vi "HexConvert.vi"(8 "E Field":string[](array[string]), 9 "Phase Field":string[](array[string]), 10 "Pockels_Galvo_Params":T1, 11 "Frequency Record":T2) -> (2 "Interrupted":bool, 3 "Hex":string)   [LabVIEW 2017]
uses:
  Controls/Frequency Record.ctl
  Controls/Pockels_Galvo_Params.ctl
  Global Variables/General Globals.vi
panel:
  out "x-y":u32
  out "Numeric":i32
  # "RE-ENTRANT"
  # "SUBROUTINE"
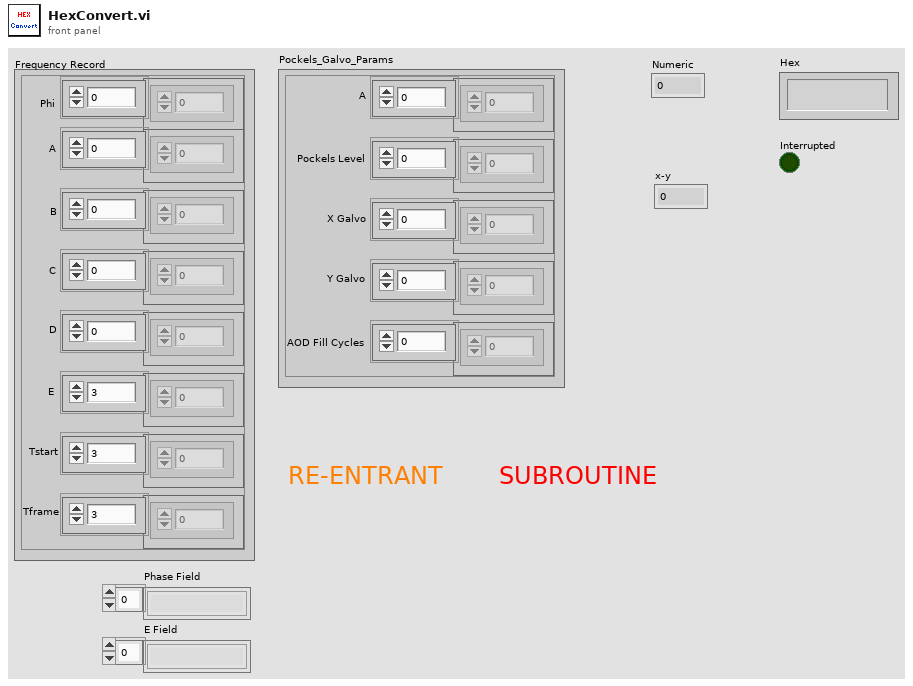
[diagram p1: front panel]
types:
  T1 = typedef "Pockels_Galvo_Params.ctl" = cluster{"A":dbl[], "Pockels Level":dbl[], "X Galvo":dbl[], "Y Galvo":dbl[], "AOD Fill Cycles":dbl[]}
  T2 = typedef "Frequency Record.ctl" = cluster{"Phi":dbl[], "A":dbl[], "B":dbl[], "C":dbl[], "D":dbl[], "E":dbl[], "Tstart":dbl[], "Tframe":dbl[]}
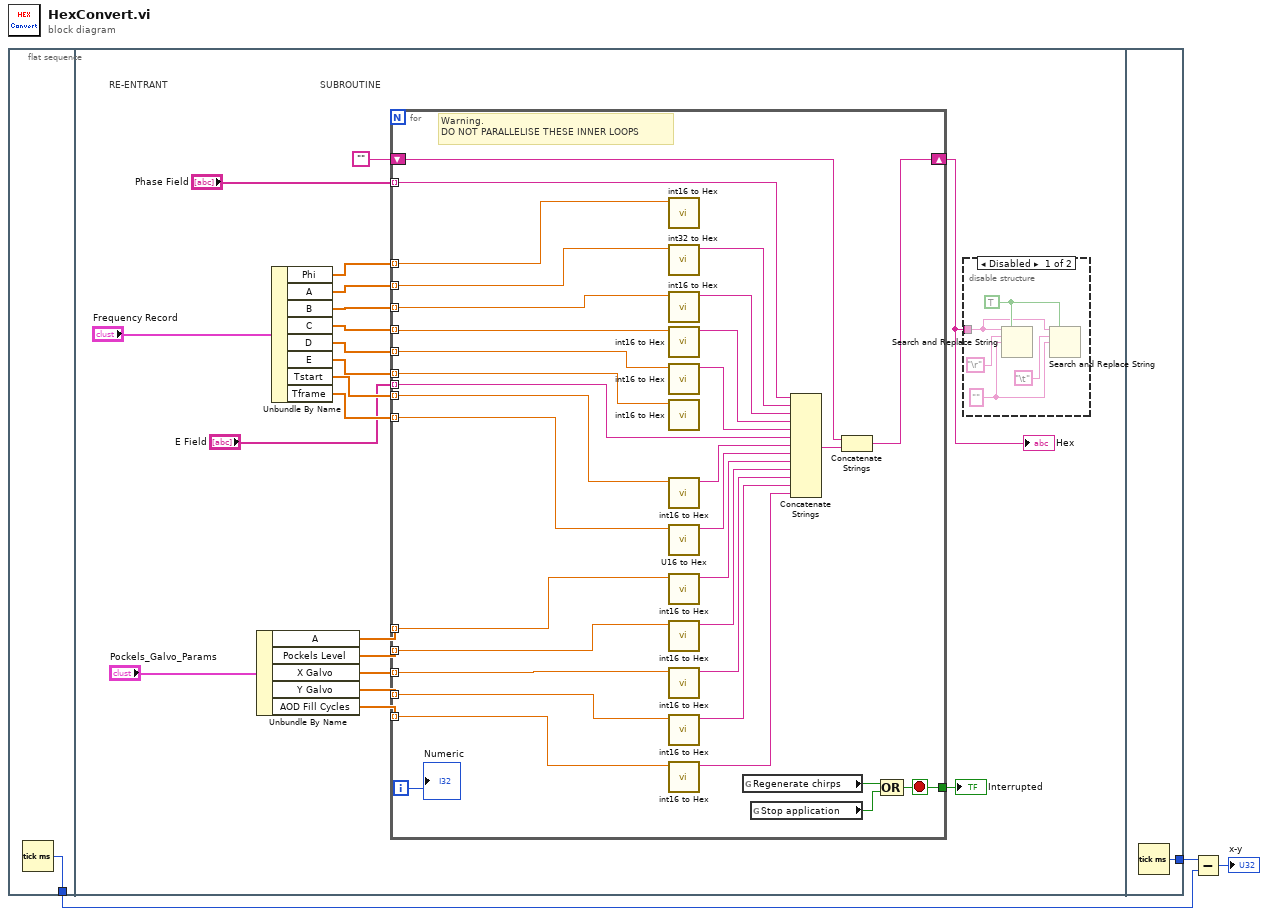
[diagram p0: block diagram]
diagram:
  n1 = flat-sequence {
    tunnel: [w4] -> w2
    tunnel: [w63] -> w3
    frame #0 {
      n2 = Tick Count (ms)() -> (millisecond timer value=w4:u32)
    }
    frame #1 {
      # "SUBROUTINE"
      # "RE-ENTRANT"
      n3 = Unbundle By Name("Pockels_Galvo_Params") -> ("A"=w23:dbl[], "Pockels Level"=w22:dbl[], "X Galvo"=w21:dbl[], "Y Galvo"=w20:dbl[], "AOD Fill Cycles"=w13:dbl[])
      n4 = Unbundle By Name("Frequency Record") -> ("Phi"=w24:dbl[], "A"=w12:dbl[], "B"=w19:dbl[], "C"=w18:dbl[], "D"=w17:dbl[], "E"=w16:dbl[], "Tstart"=w15:dbl[], "Tframe"=w14:dbl[])
      n5 = for {
        tunnel: w24 -> [w61] mode=indexing
        tunnel: w23 -> [w52] mode=indexing
        tunnel: w22 -> [w50] mode=indexing
        tunnel: w21 -> [w48] mode=indexing
        tunnel: w20 -> [w42] mode=indexing
        tunnel: w12 -> [w60] mode=indexing
        tunnel: w19 -> [w58] mode=indexing
        tunnel: w18 -> [w57] mode=indexing
        tunnel: w17 -> [w56] mode=indexing
        tunnel: w16 -> [w54] mode=indexing
        tunnel: w15 -> [w39] mode=indexing
        tunnel: w14 -> [w37] mode=indexing
        tunnel: w13 -> [w45] mode=indexing
        shift-right: [w40] -> w8
        shift-left: "" -> [w35]
        tunnel: [w32] -> w7
        tunnel: "Phase Field" -> [w31] mode=indexing
        tunnel: "E Field" -> [w30] mode=indexing
        i -> [w38]
        stop <- w32 stop-if-true
        # "Warning.\nDO NOT PARALLELISE THESE INNER LOOPS"
        n6 = call "int16 to Hex.vi"("number"=w61) -> ()  [unwired: 10 in, 1 out]
        n7 = call "int32 to Hex.vi"("number"=w60) -> ("Hex string"=w62:string)  [unwired: 10 in]
        n8 = call "int16 to Hex.vi"("number"=w58) -> ("Hex string"=w59:string)  [unwired: 10 in]
        n9 = call "int16 to Hex.vi"("number"=w57) -> ("Hex string"=w44:string)  [unwired: 10 in]
        n10 = call "int16 to Hex.vi"("number"=w56) -> ("Hex string"=w55:string)  [unwired: 10 in]
        n11 = call "int16 to Hex.vi"("number"=w54) -> ()  [unwired: 10 in, 1 out]
        n12 = call "int16 to Hex.vi"("number"=w39) -> ("Hex string"=w43:string)  [unwired: 10 in]
        n13 = call "U16 to Hex.vi"("number"=w37) -> ("Hex string"=w36:string)  [unwired: 10 in]
        n14 = call "int16 to Hex.vi"("number"=w52) -> ("Hex string"=w53:string)  [unwired: 10 in]
        n15 = call "int16 to Hex.vi"("number"=w50) -> ("Hex string"=w51:string)  [unwired: 10 in]
        n16 = call "int16 to Hex.vi"("number"=w48) -> ("Hex string"=w49:string)  [unwired: 10 in]
        n17 = call "int16 to Hex.vi"("number"=w42) -> ("Hex string"=w47:string)  [unwired: 10 in]
        n18 = call "int16 to Hex.vi"("number"=w45) -> ("Hex string"=w46:string)  [unwired: 10 in]
        n19 = global read "General Globals.vi" "Regenerate chirps"() -> (w33:bool)
        n20 = global read "General Globals.vi" "Stop application"() -> (w34:bool)
        n21 = Concatenate Strings(w31, w62, w59, w44, w55, w30, w43, w36, w53, w51, w49, w47, w46) -> (w41:string)
        n22 = Concatenate Strings(w35, w41) -> (w40:string)
        n23 = Compound Arithmetic op=OR(w33, w34) -> (w32:bool)
        "Numeric" <- w38
      }
      "Hex" <- w8
      "Interrupted" <- w7
      n24 = disable-structure shown="Disabled" {
        disable-tunnel: w8 -> [w25 _]
        frame Disabled {
          w27 = TRUE
          w26 = "" ("replace string (\"\")")
          n25 = Search and Replace String(replace all?=w27, input string=w25, search string="\r", replace string=w26) -> ()  [unwired: 4 in, 4 out]
          n26 = Search and Replace String(replace all?=w27, input string=w25, search string="\t", replace string=w26) -> ()  [unwired: 4 in, 4 out]
        }
        frame Enabled {
        }
      }
    }
    frame #2 {
      n27 = Tick Count (ms)() -> (millisecond timer value=w63:u32)
    }
  }
  n28 = Subtract(x=w3, y=w2) -> (x-y=→"x-y":u32)
